vi "Network-Get Discovery Address.vi"(7 "Address":string) -> (8 "subnet address":u32, 10 "subnet address":string)   [LabVIEW 2020]
uses:
  <vilib>/regexp/Match Regular Expression.xnode
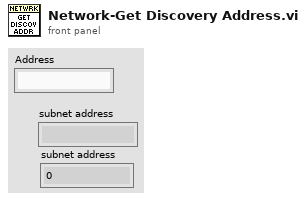
[diagram p1: front panel]
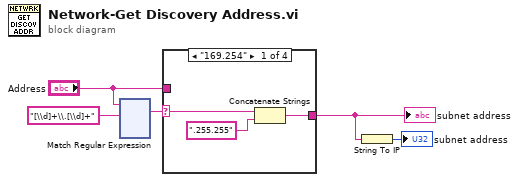
[diagram p0: block diagram]
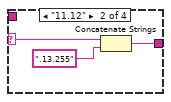
[diagram p2: hidden frame]
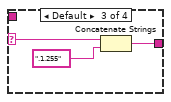
[diagram p3: hidden frame]
diagram:
  n1 = xnode "Match Regular Expression"("input string"="Address", "regular expression"="[\\d]+\\.[\\d]+") -> ("whole match"=w4:string)  [unwired: 4 in, 4 out]
  n2 = case shown="\"169.254\"" w4 {
    selector: w4 -> [w8 w11 w14 _]
    tunnel: [w6 w9 w12 w15] -> w2
    tunnel: "Address" -> [_ _ _ w15]
    frame "169.254" {
      n3 = Concatenate Strings(w8, ".255.255") -> (w6:string)
    }
    frame "11.12" {
      n4 = Concatenate Strings(w11, ".13.255") -> (w9:string)
    }
    frame Default {
      n5 = Concatenate Strings(w14, ".1.255") -> (w12:string)
    }
    frame "127.0" {
    }
  }
  "subnet address" <- w2
  n6 = String To IP(1:w2) -> (0:→"subnet address":u32)
